vi "Untitled 6 (SubVI).vi"(8 "error in":errorcluster, 9 "Numeric":i32, 10 "Array 2":T1(array[cluster]), 11 "Array":refnum<file>[](array[refnum])) -> (0 "error out":errorcluster, 3 "Array 3":refnum<file>[](array[refnum]))   [LabVIEW 2015]
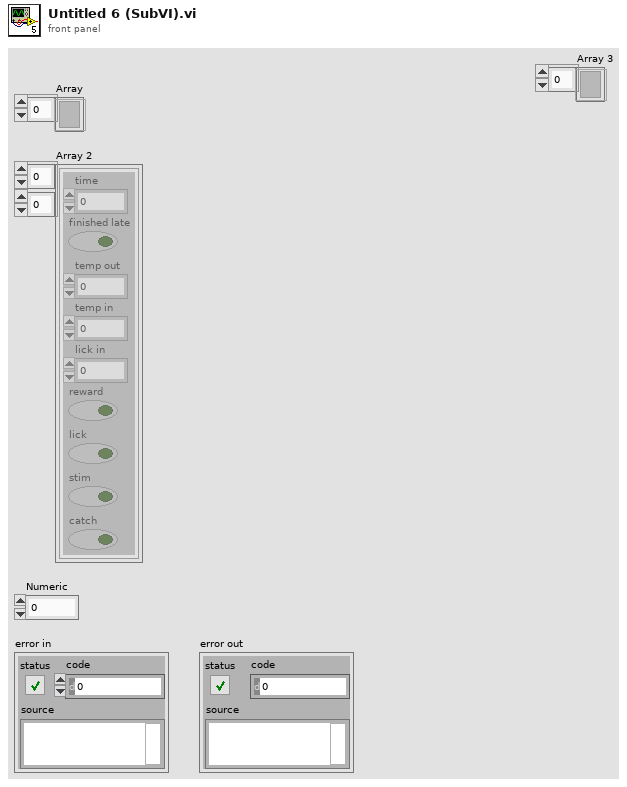
[diagram p1: front panel]
types:
  T1 = cluster{"time":u32, "finished late":bool, "temp out":sgl, "temp in":sgl, "lick in":sgl, "reward":bool, "lick":bool, "stim":bool, "catch":bool}[][]
  T2 = cluster{"time":u32, "finished late":bool, "temp out":sgl, "temp in":sgl, "lick in":sgl, "reward":bool, "lick":bool, "stim":bool, "catch":bool}[]
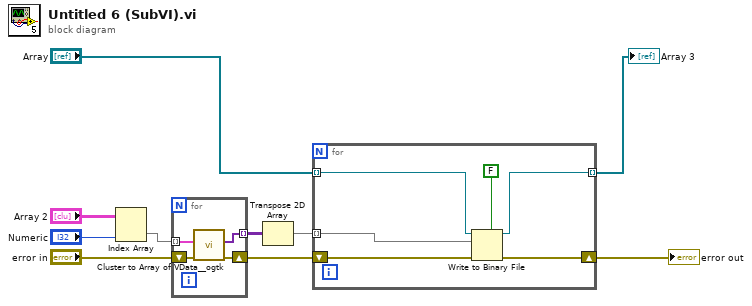
[diagram p0: block diagram]
diagram:
  n1 = Index Array(array="Array 2", index (col)="Numeric") -> (element=w8:T2)  [unwired: 1 in]
  n2 = for {
    tunnel: w8 -> [w14] mode=indexing
    tunnel: [w13] -> w7 mode=indexing
    shift-right: [w11] -> w3
    shift-left: "error in" -> [w12]
    n3 = call <userlib>:"Cluster to Array of VData__ogtk.vi"("error in (no error)"=w12, "Cluster"=w14) -> ("error out"=w11:errorcluster, "Array of VData"=w13:variant[])  [unwired: 8 in]
  }
  n4 = Transpose 2D Array(2D array=w7) -> (transposed array=w6:variant[][])
  n5 = for {
    tunnel: w6 -> [w15] mode=indexing
    tunnel: "Array" -> [w19] mode=indexing
    tunnel: [w18] -> w4 mode=indexing
    shift-right: [w17] -> w1
    shift-left: w3 -> [w16]
    n6 = Write to Binary File(file (use dialog)=w19, data=w15, error in=w16, 5:FALSE) -> (refnum out=w18:refnum<file>, error out=w17:errorcluster)  [unwired: 2 in, 1 out]
  }
  "error out" <- w1
  "Array 3" <- w4
